vi "SynapseAPI-Get Parameter Value (I32).vi"(0 "URL":string="http://localhost:24414", 5 "Gizmo":string, 7 "Parameter":string, 11 "error in (no error)":errorcluster) -> (8 "value":i32, 15 "error out":errorcluster)   [LabVIEW 2020]
uses:
  <vilib>/httpClient/LabVIEWHTTPClient.lvlib
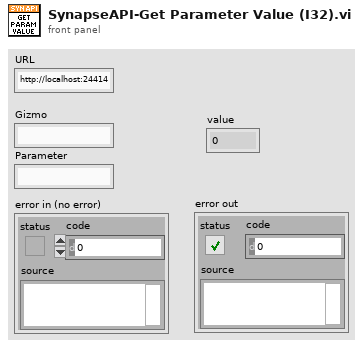
[diagram p1: front panel]
types:
  T1 = typedef "LabVIEWHTTPClient.lvlib/ClientHandle.ctl" = refnum<k1>
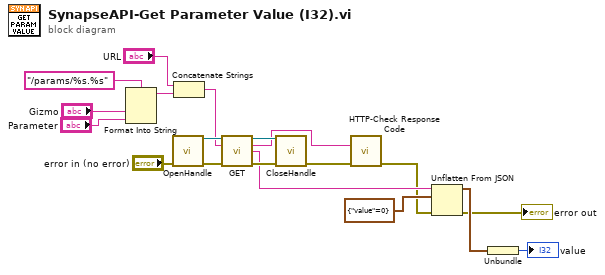
[diagram p0: block diagram]
diagram:
  n1 = Format Into String(format string="/params/%s.%s", "Gizmo", "Parameter") -> (resulting string=w9:string)  [unwired: 2 in, 1 out]
  n2 = call <vilib>:"OpenHandle.vi"("error in (no error)"="error in (no error)") -> ("client handle out"=w17:T1, "error out"=w16:errorcluster)  [unwired: 13 in]
  n3 = Concatenate Strings("URL", w9) -> (w11:string)
  n4 = call <vilib>:"GET.vi"("client handle"=w17, "url"=w11, "error in (no error)"=w16) -> ("client handle out"=w18:T1, "headers"=w2:string, "body"=w14:string, "error out"=w19:errorcluster)  [unwired: 9 in]
  n5 = call <vilib>:"CloseHandle.vi"("client handle"=w18, "error in (no error)"=w19) -> ("error out"=w3:errorcluster)  [unwired: 13 in]
  n6 = call "HTTP-Check Response Code.vi"("headers"=w2, "error in"=w3) -> ("error out"=w1:errorcluster)  [unwired: 13 in]
  n7 = Unflatten From JSON(JSON string=w14, type and defaults=cluster{"value":i32} {"value"=0} ("Cluster"), error in (no error)=w1) -> (value=w12:cluster{"value":i32}, error out=→"error out":errorcluster)  [unwired: 4 in]
  n8 = Unbundle(w12) -> ("value"=→"value":i32)
